vi "N664CW.vi"(4 "Special Function In":string, 6 "Velocity":dbl, 7 "Abort":bool, 8 "Axis":bool[](array[boolean]), 9 "Positions":dbl[](array[numeric]), 10 "Action":T1=enum."MVR", 11 "VISA In":refnum<visa-resource-name>) -> (0 "Special Function":string, 1 "Status":bool, 2 "Position Out":dbl[](array[numeric]), 3 "VISA Out":refnum<visa-resource-name>)   [LabVIEW 2014]
uses:
  Controls/StageStates.ctl
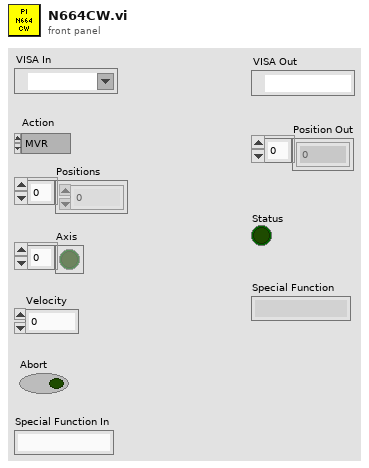
[diagram p1: front panel]
types:
  T1 = typedef "StageStates.ctl" = enum16{"POSITION", "MVR", "MOVE", "HALT", "ONTARGET", "ERROR", "EXIT", "HOME", "ZEROPOS", "NANOPOS", "QUIT", "ANALOG"}
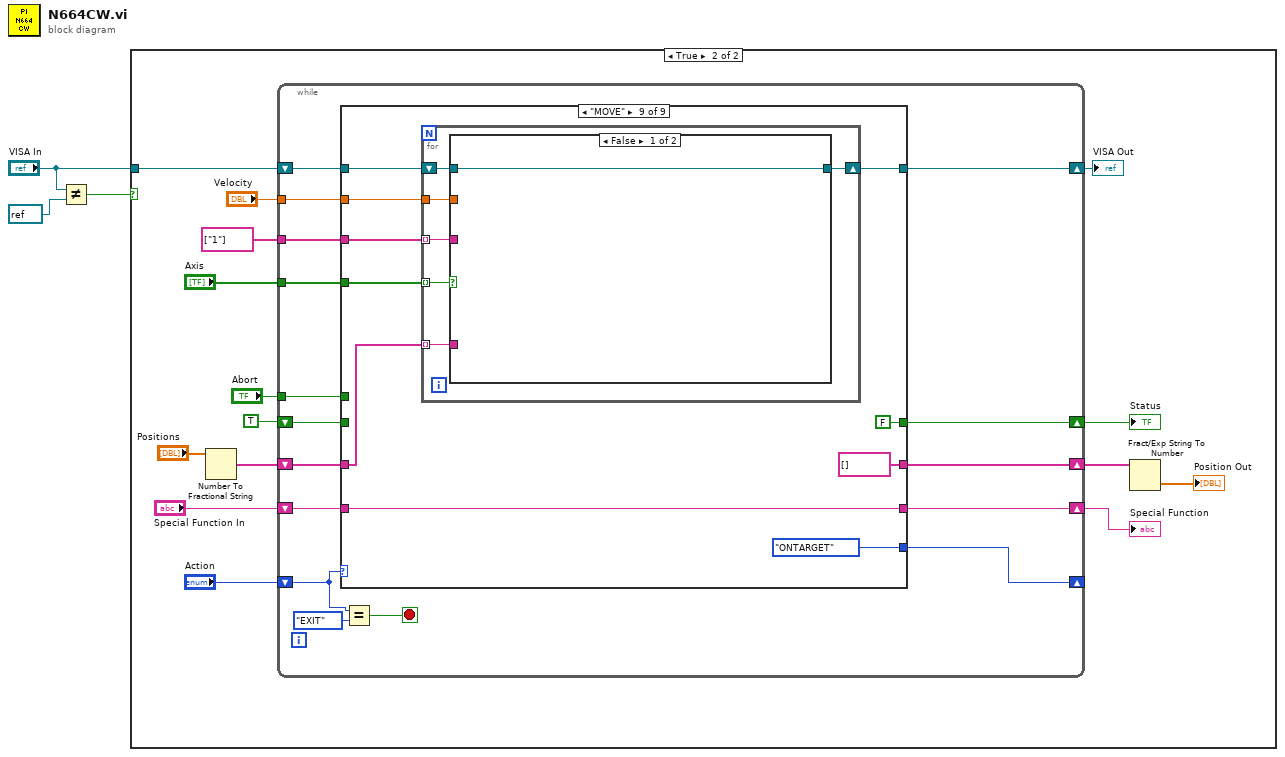
[diagram p0: block diagram]
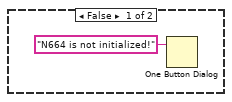
[diagram p2: hidden frame]
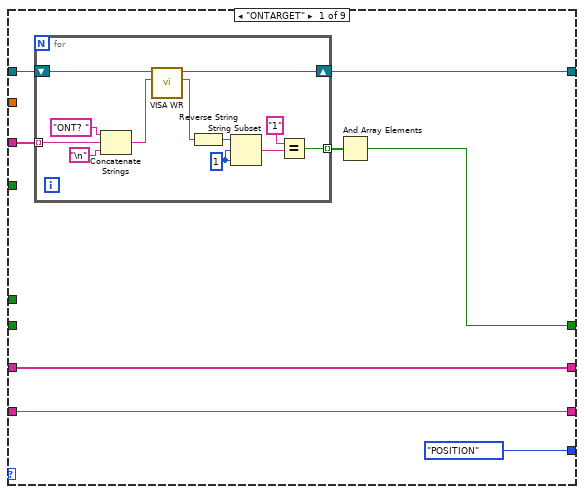
[diagram p3: hidden frame]
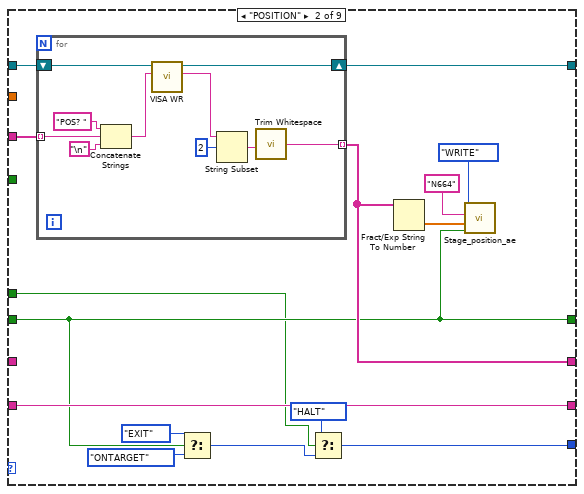
[diagram p4: hidden frame]
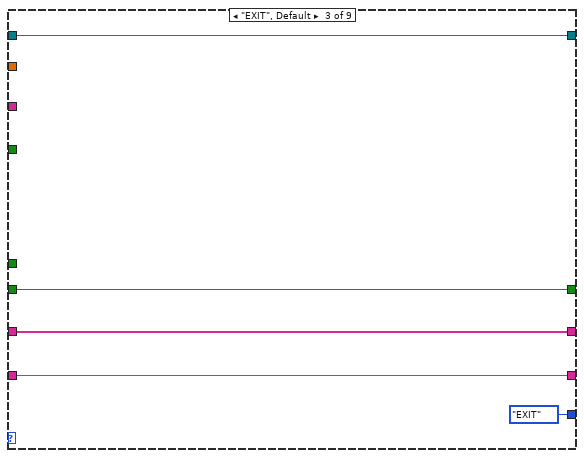
[diagram p5: hidden frame]
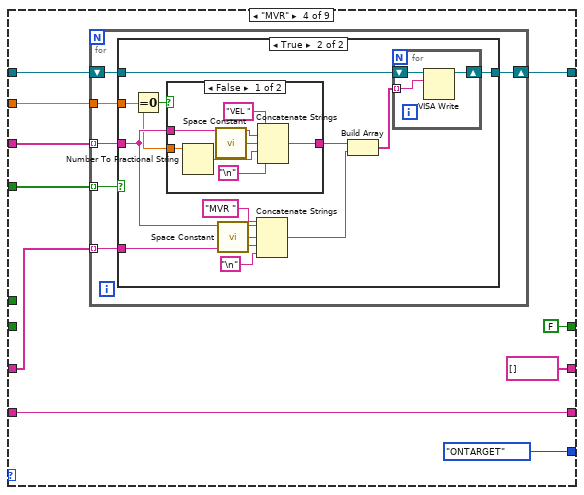
[diagram p6: hidden frame]
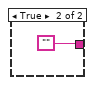
[diagram p8: hidden frame]
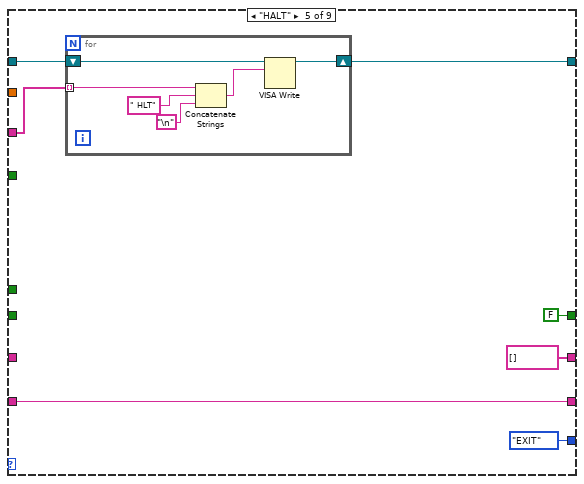
[diagram p9: hidden frame]
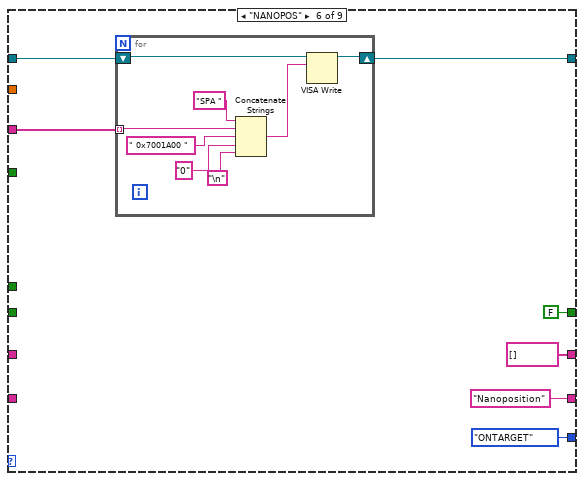
[diagram p10: hidden frame]
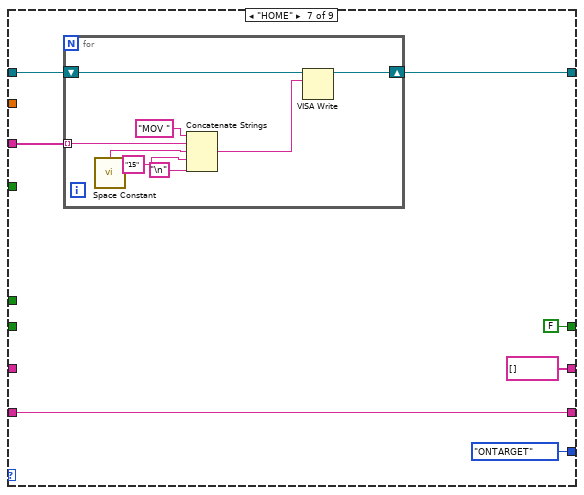
[diagram p11: hidden frame]
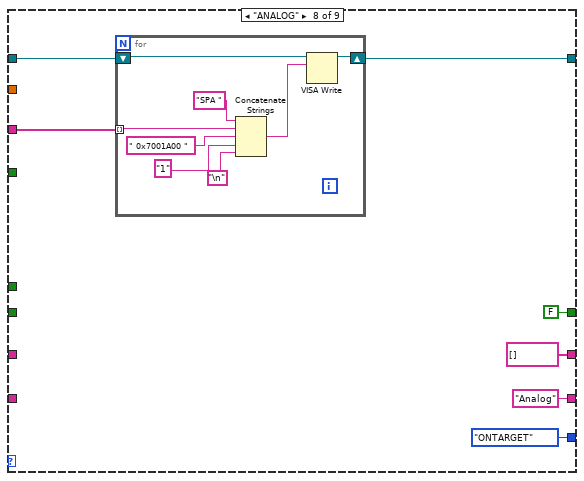
[diagram p12: hidden frame]
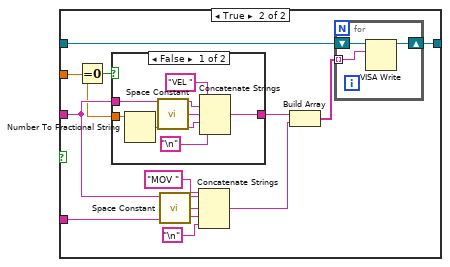
[diagram p13: hidden frame]
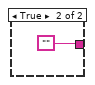
[diagram p14: hidden frame]
diagram:
  n1 = Not Equal?(x="VISA In", y=refnum<visa-resource-name> refnum ("VISA In")) -> (x != y?=w1:bool)
  n2 = case shown="True" w1 {
    tunnel: "VISA In" -> [_ w19]
    frame False {
      n3 = One Button Dialog(message="N664 is not initialized!") -> ()  [unwired: 1 in, 1 out]
    }
    frame True {
      n4 = Number To Fractional String(number="Positions") -> (F-format string=w13:string[])  [unwired: 3 in]
      n5 = while {
        tunnel: string[] ["1"] -> [w35]
        shift-right: [w25] -> _
        shift-left: "Action" -> [w29]
        shift-right: [w32] -> w12
        shift-left: w13 -> [w33]
        shift-right: [w30] -> w17
        shift-left: TRUE -> [w31]
        tunnel: "Axis" -> [w28]
        tunnel: "Velocity" -> [w26]
        shift-right: [w23] -> w9
        shift-left: "Special Function In" -> [w24]
        shift-right: [w21] -> w6
        shift-left: w19 -> [w34]
        tunnel: "Abort" -> [w20]
        stop <- w22 stop-if-true
        n6 = case shown="\"MOVE\"" w29 {
          tunnel: w35 -> [w42 w69 _ w94 w132 w144 w160 w174 w192]
          tunnel: w34 -> [w43 w70 w85 w95 w131 w145 w159 w175 w193]
          tunnel: w33 -> [w40 _ w83 w93 _ _ _ _ w191]
          tunnel: [w40 w59 w83 string[] [] string[] [] string[] [] string[] [] string[] [] string[] []] -> w32
          tunnel: w31 -> [_ w57 w84 _ _ _ _ _ _]
          tunnel: [w38 w57 w84 FALSE FALSE FALSE FALSE FALSE FALSE] -> w30
          tunnel: w28 -> [_ _ _ w92 _ _ _ _ w190]
          tunnel: w26 -> [_ _ _ w91 _ _ _ _ w189]
          tunnel: [StageStates."POSITION" ("Action") w58 StageStates."EXIT" ("Action") StageStates."ONTARGET" ("Action") StageStates."EXIT" ("Action") StageStates."ONTARGET" ("Action") StageStates."ONTARGET" ("Action") StageStates."ONTARGET" ("Action") StageStates."ONTARGET" ("Action")] -> w25
          tunnel: w24 -> [w39 w68 w82 w89 w130 _ w158 _ w188]
          tunnel: [w39 w68 w82 w89 w130 "Nanoposition" w158 "Analog" w188] -> w23
          tunnel: [w37 w67 w85 w88 w128 w141 w154 w169 w187] -> w21
          tunnel: w20 -> [_ w56 _ _ _ _ _ _ _]
          frame "ONTARGET" {
            n7 = for {
              tunnel: w42 -> [w54] mode=indexing
              tunnel: [w50] -> w41 mode=indexing
              shift-right: [w44] -> w37
              shift-left: w43 -> [w55]
              w46 = 1 ("length (rest)")
              n8 = Concatenate Strings("ONT? " ("string"), w54, "\n") -> (w45:string)
              n9 = call "VISA WR.vi"("write buffer"=w45, "VISA Refnum in"=w55) -> ("read buffer"=w53:string, "VISA Refnum out"=w44:refnum<visa-resource-name>)  [unwired: 7 in, 1 out]
              n10 = Reverse String(1:w53) -> (0:w47:string)
              n11 = String Subset(string=w47, offset (0)=w46, length (rest)=w46) -> (substring=w52:string)
              n12 = Equal?(x="1", y=w52) -> (x = y?=w50:bool)
            }
            n13 = And Array Elements(Boolean array=w41) -> (logical AND=w38:bool)
          }
          frame "POSITION" {
            n14 = for {
              tunnel: w69 -> [w79] mode=indexing
              tunnel: [w77] -> w59 mode=indexing
              shift-right: [w71] -> w67
              shift-left: w70 -> [w80]
              n15 = Concatenate Strings("POS? " ("string"), w79, "\n") -> (w72:string)
              n16 = call "VISA WR.vi"("write buffer"=w72, "VISA Refnum in"=w80) -> ("read buffer"=w78:string, "VISA Refnum out"=w71:refnum<visa-resource-name>)  [unwired: 7 in, 1 out]
              n17 = String Subset(string=w78, offset (0)=2) -> (substring=w73:string)  [unwired: 1 in]
              n18 = call <vilib>:"Trim Whitespace.vi"("string"=w73) -> ("trimmed string"=w77:string)  [unwired: 1 in]
            }
            n19 = Select(t=StageStates."EXIT" ("Action"), s=w57, f=StageStates."ONTARGET" ("Action")) -> (s? t:f=w65:T1)
            n20 = Select(t=StageStates."HALT", s=w56, f=w65) -> (s? t:f=w58:T1)
            n21 = Fract/Exp String To Number(string=w59) -> (number=w60:dbl[])  [unwired: 3 in, 1 out]
            n22 = call "Stage_position_ae.vi"("Status In"=w57, "Position In"=w60, "StageID"="N664", "Enum"=enum16{"WRITE", "READ"}."WRITE") -> ()  [unwired: 6 in, 2 out]
          }
          frame "EXIT", Default {
          }
          frame "MVR" {
            n23 = for {
              tunnel: w94 -> [w101] mode=indexing
              tunnel: w93 -> [w100] mode=indexing
              shift-right: [w98] -> w88
              shift-left: w95 -> [w99]
              tunnel: w92 -> [w97] mode=indexing
              tunnel: w91 -> [w96]
              n24 = case shown="True" w97 {
                tunnel: w101 -> [_ w108]
                tunnel: w100 -> [_ w111]
                tunnel: w99 -> [w102 w110]
                tunnel: [w102 w109] -> w98
                tunnel: w96 -> [_ w107]
                frame False {
                }
                frame True {
                  n25 = Equal To 0?(x=w107) -> (x = 0?=w106:bool)
                  n26 = case shown="False" w106 {
                    tunnel: w108 -> [w121 _]
                    tunnel: w107 -> [w118 _]
                    tunnel: [w120 ""] -> w105
                    frame False {
                      n27 = Number To Fractional String(number=w118) -> (F-format string=w119:string)  [unwired: 3 in]
                      n28 = call <vilib>:"Space Constant.vi"() -> ("String"=w124:string)
                      n29 = Concatenate Strings("VEL ", w121, w124, w119, "\n") -> (w120:string)
                    }
                    frame True {
                    }
                  }
                  n30 = call <vilib>:"Space Constant.vi"() -> ("String"=w112:string)
                  n31 = Concatenate Strings("MVR ", w108, w112, w111, "\n") -> (w104:string)
                  n32 = Build Array(w105, w104) -> (w103:string[])
                  n33 = for {
                    shift-right: [w116] -> w109
                    shift-left: w110 -> [w117]
                    tunnel: w103 -> [w115] mode=indexing
                    n34 = VISA Write(VISA resource name=w117, write buffer=w115) -> (VISA resource name out=w116:refnum<visa-resource-name>)  [unwired: 1 in, 2 out]
                  }
                }
              }
            }
          }
          frame "HALT" {
            n35 = for {
              tunnel: w132 -> [w135] mode=indexing
              shift-right: [w133] -> w128
              shift-left: w131 -> [w134]
              n36 = Concatenate Strings(w135, " HLT" ("string"), "\n") -> (w136:string)
              n37 = VISA Write(VISA resource name=w134, write buffer=w136) -> (VISA resource name out=w133:refnum<visa-resource-name>)  [unwired: 1 in, 2 out]
            }
          }
          frame "NANOPOS" {
            n38 = for {
              shift-right: [w149] -> w141
              shift-left: w145 -> [w150]
              tunnel: w144 -> [w148] mode=indexing
              n39 = Concatenate Strings("SPA " ("string"), w148, " 0x7001A00 " ("string"), "0", "\n") -> (w146:string)
              n40 = VISA Write(VISA resource name=w150, write buffer=w146) -> (VISA resource name out=w149:refnum<visa-resource-name>)  [unwired: 1 in, 2 out]
            }
          }
          frame "HOME" {
            n41 = for {
              tunnel: w160 -> [w164] mode=indexing
              shift-right: [w162] -> w154
              shift-left: w159 -> [w163]
              n42 = call <vilib>:"Space Constant.vi"() -> ("String"=w165:string)
              n43 = Concatenate Strings("MOV " ("string"), w164, w165, "15" ("string"), "\n") -> (w161:string)
              n44 = VISA Write(VISA resource name=w163, write buffer=w161) -> (VISA resource name out=w162:refnum<visa-resource-name>)  [unwired: 1 in, 2 out]
            }
          }
          frame "ANALOG" {
            n45 = for {
              shift-right: [w179] -> w169
              shift-left: w175 -> [w180]
              tunnel: w174 -> [w178] mode=indexing
              n46 = Concatenate Strings("SPA " ("string"), w178, " 0x7001A00 " ("string"), "1", "\n") -> (w177:string)
              n47 = VISA Write(VISA resource name=w180, write buffer=w177) -> (VISA resource name out=w179:refnum<visa-resource-name>)  [unwired: 1 in, 2 out]
            }
          }
          frame "MOVE" {
            n48 = for {
              tunnel: w192 -> [w199] mode=indexing
              tunnel: w191 -> [w198] mode=indexing
              shift-right: [w196] -> w187
              shift-left: w193 -> [w197]
              tunnel: w190 -> [w195] mode=indexing
              tunnel: w189 -> [w194]
              n49 = case shown="False" w195 {
                tunnel: w199 -> [_ w206]
                tunnel: w198 -> [_ w209]
                tunnel: w197 -> [w200 w208]
                tunnel: [w200 w207] -> w196
                tunnel: w194 -> [_ w205]
                frame False {
                }
                frame True {
                  n50 = Equal To 0?(x=w205) -> (x = 0?=w204:bool)
                  n51 = case shown="False" w204 {
                    tunnel: w206 -> [w219 _]
                    tunnel: w205 -> [w216 _]
                    tunnel: [w218 ""] -> w203
                    frame False {
                      n52 = Number To Fractional String(number=w216) -> (F-format string=w217:string)  [unwired: 3 in]
                      n53 = call <vilib>:"Space Constant.vi"() -> ("String"=w222:string)
                      n54 = Concatenate Strings("VEL ", w219, w222, w217, "\n") -> (w218:string)
                    }
                    frame True {
                    }
                  }
                  n55 = call <vilib>:"Space Constant.vi"() -> ("String"=w210:string)
                  n56 = Concatenate Strings("MOV ", w206, w210, w209, "\n") -> (w202:string)
                  n57 = Build Array(w203, w202) -> (w201:string[])
                  n58 = for {
                    shift-right: [w214] -> w207
                    shift-left: w208 -> [w215]
                    tunnel: w201 -> [w213] mode=indexing
                    n59 = VISA Write(VISA resource name=w215, write buffer=w213) -> (VISA resource name out=w214:refnum<visa-resource-name>)  [unwired: 1 in, 2 out]
                  }
                }
              }
            }
          }
        }
        n60 = Equal?(x=w29, y=StageStates."EXIT") -> (x = y?=w22:bool)
      }
      "Status" <- w17
      "Special Function" <- w9
      "VISA Out" <- w6
      n61 = Fract/Exp String To Number(string=w12) -> (number=→"Position Out":dbl[])  [unwired: 3 in, 1 out]
    }
  }
